vi "image display probe.vi"(10 "Image Pixels (I16)":i16[][](array[numeric])) -> ()   [LabVIEW 2012]
doc: "SciScan 1.2 160622"
panel:
  out "size(s)":i32[](array[numeric])
  out "Image":T1(plugin-control)
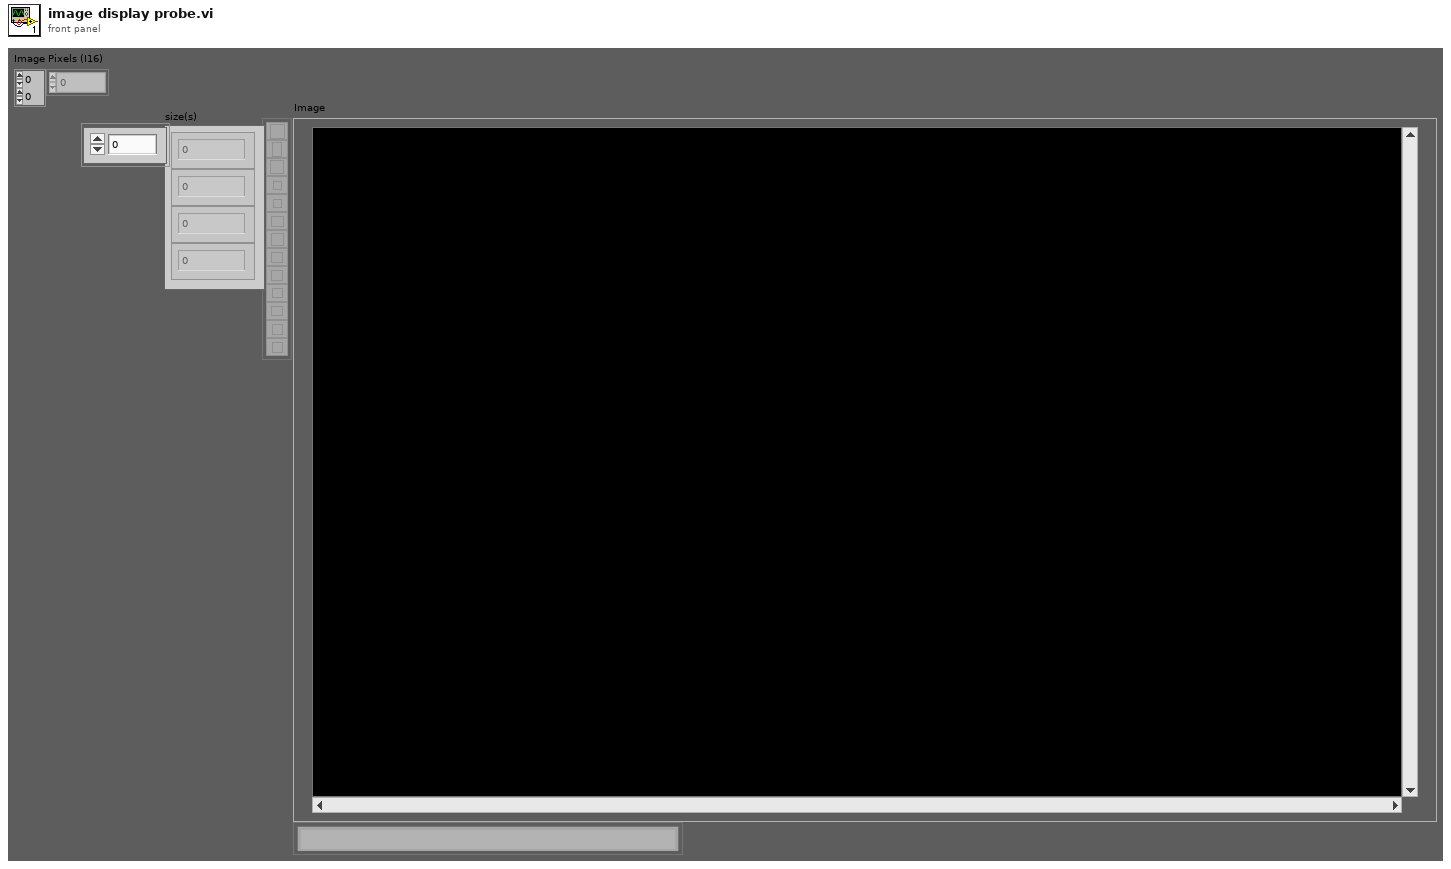
[diagram p1: front panel]
types:
  T1 = typedef "IMAQ Image.ctl" = refnum<image>
  T2 = typedef "Image Type" = u32
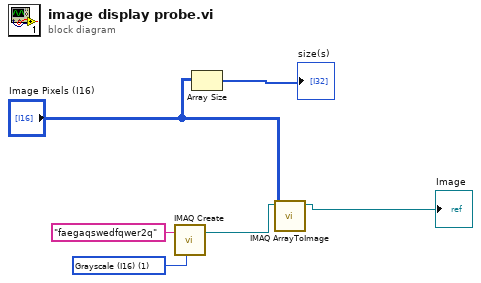
[diagram p0: block diagram]
diagram:
  w5 = T2 1 items=["Grayscale (U8)", "Grayscale (I16)", "Grayscale (SGL)", "Complex (CSG)", "RGB (U32)", "HSL (U32)", "RGB (U64)", "Grayscale (U16)"] ("Image Type")
  n1 = call "IMAQ Create"("Image Name"="faegaqswedfqwer2q", "Image Type"=w5) -> ("New Image"=w4:T1)  [unwired: 3 in, 1 out]
  n2 = Array Size(array="Image Pixels (I16)") -> (size(s)=→"size(s)":i32[])
  n3 = call "IMAQ ArrayToImage"("Image Pixels (I16)"="Image Pixels (I16)", "Image"=w4) -> ("Image Out"=→"Image":T1)  [unwired: 8 in, 1 out]
